vi "zrotg - Givens Rotation Parameters (CDB).vi"(10 "y":cdb, 11 "x":cdb) -> (0 "error":i32, 2 "s":cdb, 3 "c":dbl, 4 "z":cdb, 5 "r":cdb)   [LabVIEW 2018, in "NI_AALBLAS.lvlib"]
doc: "Creates the parameters used in the rot - Givens Rotation VI."
uses:
  NI_AALBLAS.lvlib
  <resource>/lvblas.dll
panel:
  # "{"
  # "-"
  # "-s*x+c*y=0"
  # "c*x+s*y=r"
  # "c +|s| =1"
  # "2"
  # "2"
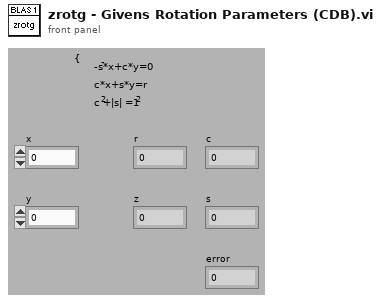
[diagram p1: front panel]
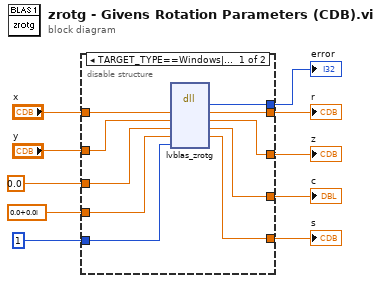
[diagram p0: block diagram]
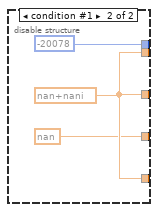
[diagram p2: hidden frame]
diagram:
  n1 = disable-structure shown="TARGET_TYPE==Windows||TARGET_TYPE==Unix||TARGET_TYPE==RT||TARGET_TYPE==Mac" {
    disable-tunnel: [w20 -20078] -> w10
    disable-tunnel: [w19 w22] -> w7
    disable-tunnel: [w18 w22] -> w6
    disable-tunnel: "x" -> [w17 _]
    disable-tunnel: "y" -> [w16 _]
    disable-tunnel: [w15 nan] -> w5
    disable-tunnel: [w14 w22] -> w4
    disable-tunnel: 0.0 -> [w13 _]
    disable-tunnel: cdb 0.0+0.0i -> [w12 _]
    disable-tunnel: 1 -> [w11 _]
    frame condition #0 (active) {
      n2 = dll-call lib="C:/Program Files (x86)/National Instruments/LabVIEW 2018/resource/lvblas.*" fn="lvblas_zrotg" ("CBLAS.dll:DotProdH")("x"=w17, "y"=w16, "c"=w13, "s"=w12, "check"=w11) -> ("error"=w20:i32, "x"=w19:cdb, "y"=w18:cdb, "c"=w15:dbl, "s"=w14:cdb)  [unwired: 4 in, 2 out]
    }
    frame condition #1 {
      w22 = cdb nan+nani
    }
  }
  "error" <- w10
  "c" <- w5
  "s" <- w4
  "r" <- w7
  "z" <- w6
